vi "Upload to Sift Async.vi"(7 "Absolute Filepath":path, 8 "Run Name":string="TDMS Upload Example", 9 "Asset Name":string="LabVIEW-TDMS-Example", 10 "API Key":string, 11 "API URL":string) -> ()   [LabVIEW 2024, in "Sift TDMS Uploader.lvlib" / "Sift TDMS Uploader.lvclass"]
uses:
  Sift TDMS Uploader.lvclass
  Upload to Sift.vi
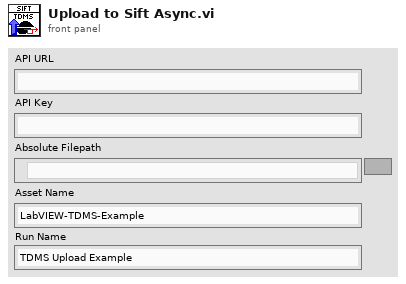
[diagram p1: front panel]
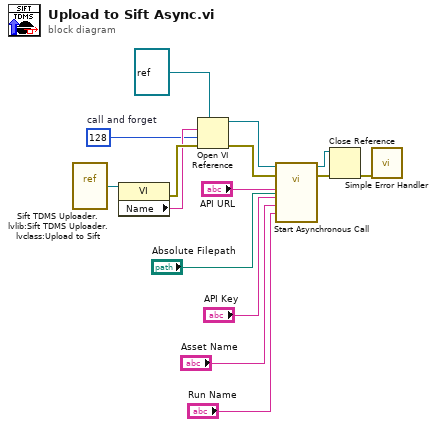
[diagram p0: block diagram]
diagram:
  w6 = 128  # call and forget
  n1 = vi-ref "Sift TDMS Uploader.lvlib:Sift TDMS Uploader.lvclass:Upload to Sift.vi"() -> (w13:refnum<vi>)
  n2 = property class="VI"(reference=w13) -> (error out=w15:errorcluster, "Name"=w14:string)  [unwired: 1 in, 1 out]
  n3 = Open VI Reference(type specifier VI Refnum (for type only)=refnum<vi> refnum, vi path=w14, options=w6, error in (no error)=w15) -> (vi reference=w8:refnum<vi>, error out=w9:errorcluster)  [unwired: 2 in]
  n4 = call-by-ref "Start Asynchronous Call"(reference=w8, error in=w9, "Absolute Filepath"="Absolute Filepath", "Run Name"="Run Name", "Asset Name"="Asset Name", "API Key"="API Key", "API URL"="API URL") -> (reference out=w11:refnum<vi>, error out=w10:errorcluster)  [unwired: 6 in, 1 out]
  n5 = Close Reference(reference=w11, error in (no error)=w10) -> (error out=w12:errorcluster)
  n6 = call <vilib>:"Simple Error Handler.vi"("error in (no error)"=w12) -> ()  [unwired: 4 in, 5 out]
